vi "GetEnvelopeCoords.vi"(0 "Servo Min":T1, 5 "Empty initialized Array in":dbl[][](array[numeric]), 7 "L2":dbl, 9 "L1":dbl, 11 "origin in":cluster{"x":i16, "y":i16}={"x"=200, "y"=200}) -> (1 "theta1":dbl=179.0, 2 "Servo Max":T1={"servo 1"=180.0, "servo 2"=180.0, "servo 3"=0.0}, 3 "theta3":dbl=-358.0, 4 "theta2":dbl=179.0, 6 "In Range?":bool, 8 "y2":dbl, 10 "x2":dbl, 14 "origin out":cluster{"x":i16, "y":i16}, 15 "Empty initialized Array out":dbl[][](array[numeric]))   [LabVIEW 2024]
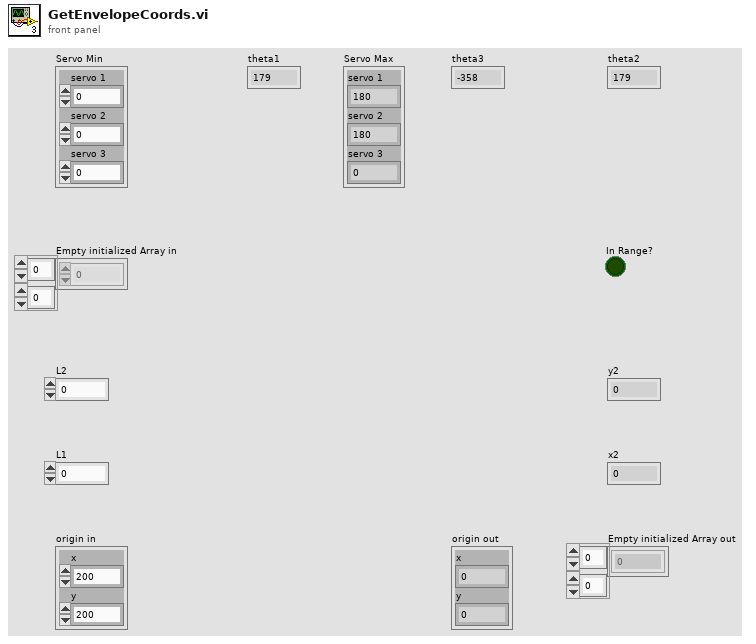
[diagram p1: front panel]
types:
  T1 = cluster{"servo 1":dbl, "servo 2":dbl, "servo 3":dbl}
  T2 = cluster{"servo 1":dbl, "servo 2":dbl, "servo 2":dbl}
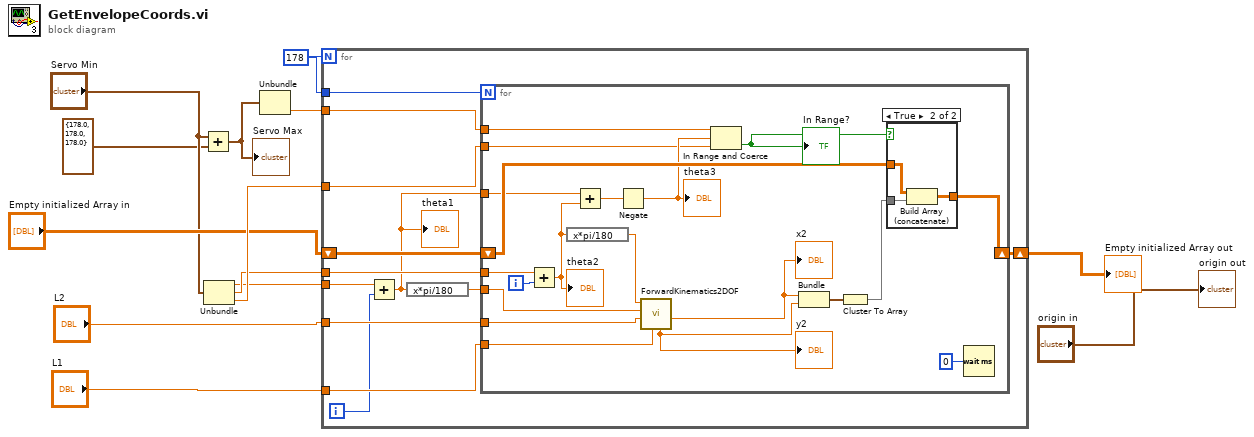
[diagram p0: block diagram]
diagram:
  w5 = 178
  n1 = Add(x="Servo Min", y=T2 {"servo 1"=178.0, "servo 2"=178.0, "servo 2"=178.0}) -> (x+y=w10:cluster{"servo 1":dbl, "servo 2":dbl, dbl})
  "Servo Max" <- w10
  n2 = Unbundle("Servo Min") -> ("servo 1"=w3:dbl, "servo 2"=w6:dbl, "servo 3"=w9:dbl)
  n3 = Unbundle(w10) -> (w11:dbl)  [unwired: 2 out]
  n4 = for {
    N: w5 -> [_]
    tunnel: "L1" -> [w24]
    tunnel: "L2" -> [w25]
    tunnel: w3 -> [w23]
    shift-right: [w21] -> w7
    shift-left: "Empty initialized Array in" -> [w22]
    tunnel: w5 -> [w20]
    tunnel: w6 -> [w18]
    tunnel: w9 -> [w16]
    tunnel: w11 -> [w15]
    i -> [w19]
    n5 = Add(x=w23, y=w19) -> (x+y=w14:dbl)
    "theta1" <- w14
    n6 = expression code="x*pi/180"(w14) -> (w17:dbl)
    n7 = for {
      N: w20 -> [_]
      tunnel: w25 -> [w38]
      tunnel: w24 -> [w45]
      tunnel: w17 -> [w36]
      shift-right: [w32] -> w21
      shift-left: w22 -> [w34]
      tunnel: w18 -> [w43]
      tunnel: w16 -> [w30]
      tunnel: w15 -> [w29]
      tunnel: w14 -> [w27]
      i -> [w42]
      n8 = Add(x=w43, y=w42) -> (x+y=w26:dbl)
      "theta2" <- w26
      n9 = expression code="x*pi/180"(w26) -> (w37:dbl)
      n10 = Add(x=w27, y=w26) -> (x+y=w35:dbl)
      n11 = Negate(x=w35) -> (-x=w31:dbl)
      "theta3" <- w31
      n12 = call "ForwardKinematics2DOF.vi"("L1"=w45, "L2"=w38, "theta1"=w36, "theta2"=w37) -> ("x2"=w40:dbl, "y2"=w41:dbl)  [unwired: 4 in, 2 out]
      "y2" <- w41
      "x2" <- w40
      n13 = In Range and Coerce(upper limit=w29, x=w31, lower limit=w30) -> (In Range?=w28:bool)  [unwired: 1 out]
      "In Range?" <- w28
      n14 = Bundle("x2"=w40, "y2"=w41) -> (w44:cluster{"x2":dbl, "y2":dbl})  [unwired: 1 in]
      n15 = Cluster To Array(cluster=w44) -> (array=w33:dbl[])
      n16 = case shown="True" w28 {
        tunnel: w34 -> [w46 w49]
        tunnel: w33 -> [_ w48]
        tunnel: [w46 w47] -> w32
        frame False {
        }
        frame True {
          n17 = Build Array (concatenate)(w49, w48) -> (w47:dbl[][])
        }
      }
      n18 = Wait (ms)(milliseconds to wait=u32 0) -> ()  [unwired: 1 out]
    }
  }
  "Empty initialized Array out" <- w7
  "origin out" <- "origin in"
